vi "Generate continuous signal.vi"() -> ()   [LabVIEW 2010]
doc: "This example shows how to program Red Pitaya to generate analog 2kHz sine wave signal with 1V amplitude. Red Pitaya is able to generate signals in range from DC to 50 MHz with output voltage range from -1 to 1 Volt. Generated signal can be observed by Red Pitaya Oscilloscope WEB application. To run it, just open web browser, input Red Pitaya IP and start Oscilloscope."
uses:
  RedPitaya.lvlib
panel:
  in  "Duty Cycle":i32=-1 min=-1 max=100
  in  "Phase":i32=361
  in  "DC Offset":dbl=2.0
  in  "Frequency (1000 Hz)":i32=2000
  in  "Waveform Function":u16(ring)=1 items=["", "Sine", "Square", "Triangle", "Sawtooth UP", "Sawtooth Down", "PWM"]
  in  "Channel (1|2)":u16(ring)=1 items=["Channel 1"=1, "Channel 2"=2]
  in  "Amplitude":dbl=1.0
  in  "IP address":string="192.168.1.100"
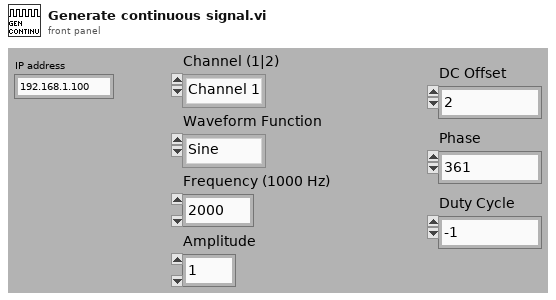
[diagram p1: front panel]
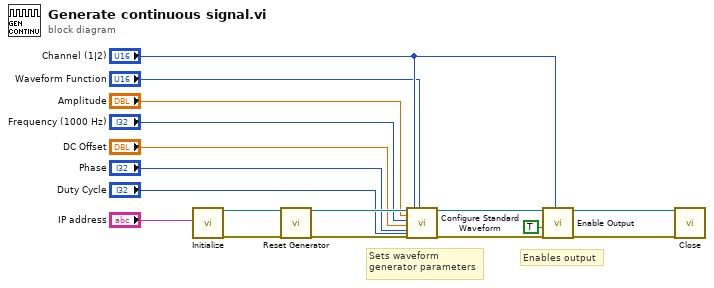
[diagram p0: block diagram]
diagram:
  # "Enables output"
  # "Sets waveform\ngenerator parameters"
  n1 = call "Initialize.vi"("IP address"="IP address") -> ("RedPitaya TCP Connection"=w11:refnum<k5>, "error out"=w8:errorcluster)  [unwired: 17 in]
  n2 = call "Reset Generator.vi"("RedPitaya connection in"=w11, "error in"=w8) -> ("RedPitaya connection out"=w10:refnum<k5>, "error out"=w9:errorcluster)  [unwired: 16 in]
  n3 = call "Configure Standard Waveform.vi"("RedPitaya connection in"=w10, "Amplitude"="Amplitude", "Frequency"="Frequency (1000 Hz)", "DC Offset"="DC Offset", "Phase"="Phase", "error in"=w9, "Channel #"="Channel (1|2)", "Duty Cycle"="Duty Cycle", "Waveform Function"="Waveform Function") -> ("RedPitaya connection out"=w15:refnum<k5>, "error out"=w14:errorcluster)  [unwired: 9 in]
  n4 = call "Enable Output.vi"("RedPitaya connection in"=w15, "Generation (T: Enable)"=TRUE, "error in"=w14, "Channel #"="Channel (1|2)") -> ("RedPitaya connection out"=w12:refnum<k5>, "error out"=w13:errorcluster)  [unwired: 14 in]
  n5 = call "Close.vi"("connection ID"=w12, "error in"=w13) -> ()  [unwired: 17 in, 1 out]
